vi "SignUp.vi"(8 "error in":errorcluster, 9 "password":string, 10 "email":string, 11 "firebase in":refnum<class "firebase.lvclass">) -> (0 "error out":errorcluster, 3 "firebase out":refnum<class "firebase.lvclass">)   [LabVIEW 2022 SP3, in "firebase.lvclass"]
uses:
  firebase.lvclass
  <vilib>/NI/Advanced HTTP Client/Header--Combo Box.ctl
  Error Message--cluster.ctl
  Success Sign In--cluster.ctl
  8df7efb1-880b-4afd-9d83-a65ebbba9a00.vi
  8b64f89a-9e96-43c3-a012-814e780b19c4.vi
  d9e4e2d6-dd7c-4b59-b05d-e984aa4a9630.vi
  <vilib>/JDP Science/JSONtext/Next JSON Value.vi
  <vilib>/JDP Science/JSONtext/String Subset.vi
  <vilib>/JDP Science/JSONtext/Parsing/Advance past next JSON Value (inlined COPY).vi
  <vilib>/JDP Science/JSONtext/Parsing/Advance past whitespace.vi
  <vilib>/JDP Science/JSONtext/Parsing/Advance past String.vi
  <vilib>/JDP Science/JSONtext/Parsing/Advance past Number.vi
  <vilib>/JDP Science/JSONtext/Parsing/Advance past Line Ending.vi
  <vilib>/JDP Science/JSONtext/Variant to JSON Text.vi
  <vilib>/NI/Advanced HTTP Client/POST (Buffer).vi
  <vilib>/JDP Science/JSONtext/Parsing/Parse Full Path or Item Name.vi
  <vilib>/JDP Science/JSONtext/Parsing/Advance past Array.vi
  <vilib>/JDP Science/JSONtext/Parsing/Advance past Object.vi
  <vilib>/JDP Science/JSONtext/support/Error Cluster From Code.vi
  <vilib>/JDP Science/JSONtext/Offset/Find Item Locations by Path.vi
  <vilib>/JDP Science/JSONtext/JSON text to Variant.vi
  <vilib>/JDP Science/JSONtext/LVClass Serializer/JSONtext LVClass Serializer.lvclass
  <vilib>/NI/Advanced HTTP Client/Session.lvclass
  <vilib>/JDP Science/JSONtext/JSONtext.lvlib
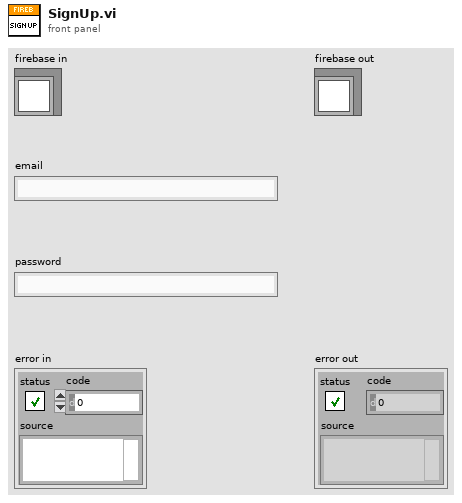
[diagram p1: front panel]
types:
  T1 = typedef "lib_NI_Advanced HTTP Client.lvlib/Session.lvclass/Header--Combo Box.ctl" = string
  T2 = cluster{"email":string, "password":string, "returnSecureToken":bool}
  T3 = typedef "firebase.lvclass/Error Message--cluster.ctl" = cluster{"error":cluster{"code":i32, "message":string, "errors":cluster{"message":string, "domain":string, "reason":string}[]}}
  T4 = typedef "firebase.lvclass/Success Sign In--cluster.ctl" = cluster{"kind":string, "idToken":string, "email":string, "refreshToken":string, "expiresIn":string, "localId":string, "displayName":string, "registered":bool}
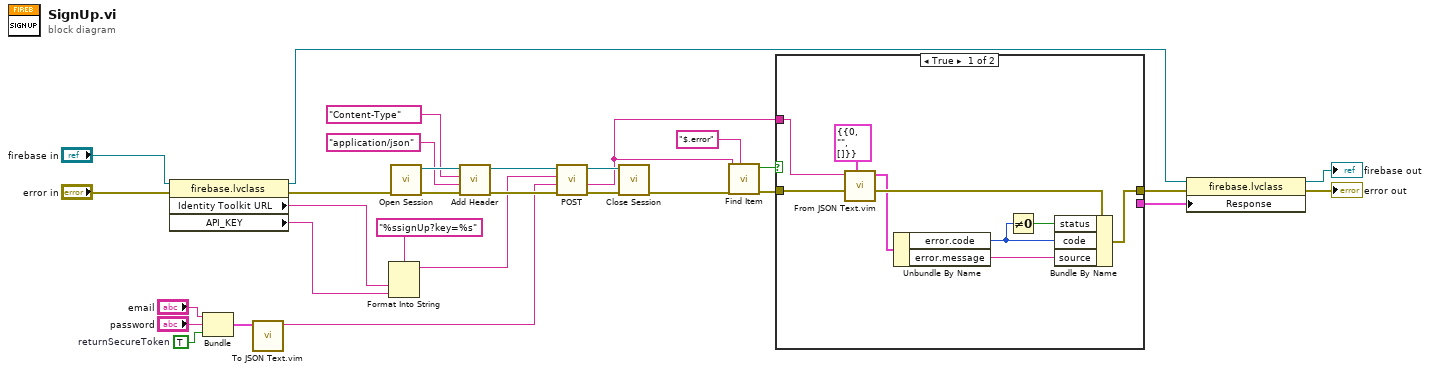
[diagram p0: block diagram]
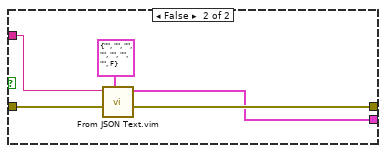
[diagram p2: hidden frame]
diagram:
  w14 = TRUE  # returnSecureToken
  n1 = property class="firebase.lvclass"(reference="firebase in", error in="error in") -> (reference out=w20:refnum<class "firebase.lvclass">, error out=w25:errorcluster, "Identity Toolkit URL"=w19:string, "API_KEY"=w17:string)
  n2 = Bundle("email"="email", "password"="password", "returnSecureToken"=w14) -> (w13:T2)  [unwired: 1 in]
  n3 = call "To JSON Text.vim"("Anything"=w13) -> ("<JSON>"=w7:string)  [unwired: 9 in, 1 out]
  n4 = Format Into String(format string="%ssignUp?key=%s", w19, w17) -> (resulting string=w6:string)  [unwired: 2 in, 1 out]
  n5 = call <vilib>:"Open Session.vi"("error in"=w25) -> ("error out"=w28:errorcluster, "session"=w11:refnum<class "Session.lvclass">)  [unwired: 9 in]
  n6 = call <vilib>:"Add Header.vi"("error in"=w28, "value"="application/json", "header"=T1 "Content-Type", "session in"=w11) -> ("error out"=w27:errorcluster, "session out"=w10:refnum<class "Session.lvclass">)  [unwired: 6 in]
  n7 = call-poly <vilib>:"POST.vi"("error in"=w27, "buffer"=w7, "url"=w6, "session in"=w10) -> ("error out"=w29:errorcluster, "body"=w3:string, "session out"=w12:refnum<class "Session.lvclass">)  [unwired: 3 in, 2 out]
  n8 = call <vilib>:"Close Session.vi"("error in"=w29, "session"=w12) -> ("error out"=w24:errorcluster)  [unwired: 9 in]
  n9 = call <vilib>:"Find Item.vi"("$Path or Item Name"="$.error", "error in (no error)"=w24, "JSON"=w3) -> ("error out"=w26:errorcluster, "Found"=w4:bool)  [unwired: 5 in, 2 out]
  n10 = case shown="True" w4 {
    tunnel: [w37 w43] -> w23
    tunnel: w26 -> [w39 w44]
    tunnel: w3 -> [w35 w42]
    tunnel: [_ w40] -> w1
    frame True {
      n11 = call "From JSON Text.vim"("Data Type and Default Value"=T3 {"error"={"code"=0, "message"="", "errors"=[]}} ("Error Message"), "error in (no error)"=w39, "JSON"=w35) -> ("error out"=w38:errorcluster, "Data out"=w34:T3)  [unwired: 7 in]
      n12 = Unbundle By Name(w34) -> ("error.code"=w33:i32, "error.message"=w31:string)
      n13 = Not Equal To 0?(x=w33) -> (x != 0?=w32:bool)
      n14 = Bundle By Name(cluster=w38, "status"=w32, "code"=w33, "source"=w31) -> (w37:errorcluster)
    }
    frame False {
      n15 = call "From JSON Text.vim"("Data Type and Default Value"=T4 {"kind"="", "idToken"="", "email"="", "refreshToken"="", "expiresIn"="", "localId"="", "displayName"="", "registered"=FALSE} ("Succes Sign In"), "error in (no error)"=w44, "JSON"=w42) -> ("error out"=w43:errorcluster, "Data out"=w40:T4)  [unwired: 7 in]
    }
  }
  n16 = property class="firebase.lvclass"(reference=w20, error in=w23, "Response"=w1) -> (reference out=→"firebase out":refnum<class "firebase.lvclass">, error out=→"error out":errorcluster)
